vi "Write Position.vi"(8 "error in (no error)":errorcluster, 10 "Position":cluster{"Left":i32, "Top":i32}, 11 "Selection in":refnum<class "Selection.lvclass">) -> (0 "error out":errorcluster, 3 "Selection out":refnum<class "Selection.lvclass">)   [LabVIEW 2015, in "LV Image Editor Framework.lvlib" / "Selection.lvclass"]
uses:
  Selection.lvclass
  Selection.lvclass/Selection.ctl
  Shape/Shape.lvclass
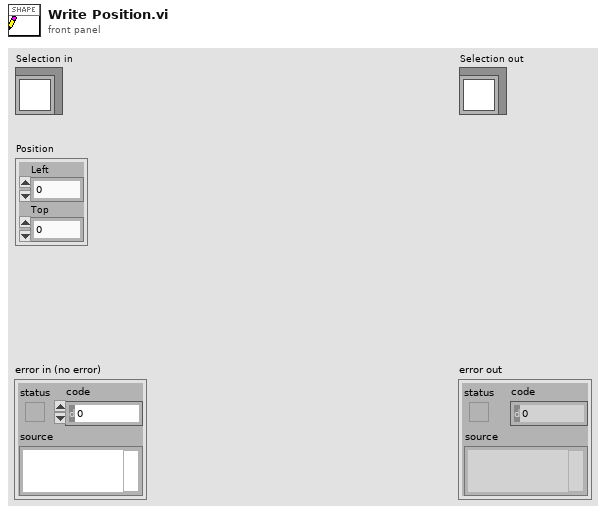
[diagram p1: front panel]
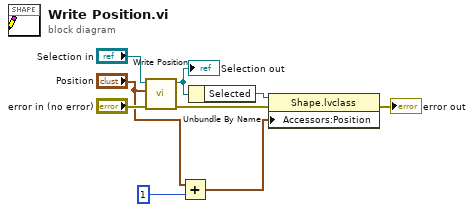
[diagram p0: block diagram]
diagram:
  n1 = call-parent "Write Position.vi"("error in (no error)"="error in (no error)", "Position"="Position", "Shape in"="Selection in") -> ("error out"=w5:errorcluster, "Shape out"=w7:refnum<class "Selection.lvclass">)  [unwired: 7 in]
  "Selection out" <- w7
  n2 = Add(x="Position", y=1) -> (x+y=w1:cluster{"Left":i32, "Top":i32})
  n3 = Unbundle By Name(w7) -> ("Selected"=w6:refnum<data-value>)
  n4 = property class="Shape.lvclass"(reference=w6, error in=w5, "Accessors:Position"=w1) -> (error out=→"error out":errorcluster)  [unwired: 1 out]
